vi "device-to-devcmd.vi"(11 "device":T2) -> (3 "dev-cmd out":T1)   [LabVIEW 2019]
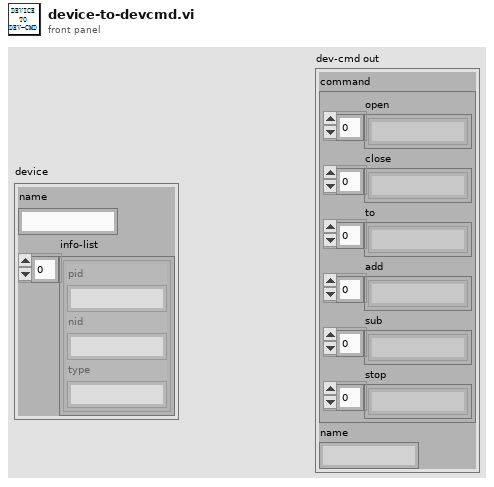
[diagram p1: front panel]
types:
  T1 = cluster{"command":cluster{"open":string[], "close":string[], "to":string[], "add":string[], "sub":string[], "stop":string[]}, "name":string}
  T2 = cluster{"name":string, "info-list":cluster{"pid":string, "nid":string, "type":string}[]}
  T3 = cluster{"pid":string, "nid":string, "type":string}[]
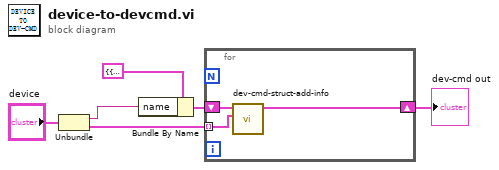
[diagram p0: block diagram]
diagram:
  n1 = Unbundle("device") -> ("name"=w2:string, "info-list"=w5:T3)
  n2 = Bundle By Name(cluster=T1 {"command"={"open"=[], "close"=[], "to"=[], "add"=[], "sub"=[], "stop"=[]}, "name"=""} ("dev-cmd out"), "name"=w2) -> (w3:T1)
  n3 = for {
    tunnel: w5 -> [w9] mode=indexing
    shift-right: [w8] -> w1
    shift-left: w3 -> [w7]
    n4 = call "dev-cmd-struct-add-info.vi"("info"=w9, "dev-cmd"=w7) -> ("dev-cmd out"=w8:T1)  [unwired: 9 in]
  }
  "dev-cmd out" <- w1
